vi "Control.AnalysisStop.vi"(11 "AnalysisRef":refnum<vi>) -> ()   [LabVIEW 2015, in "NIAnalysis.lvlib"]
uses:
  NIAnalysis.lvlib
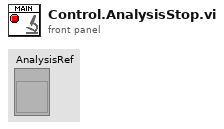
[diagram p1: front panel]
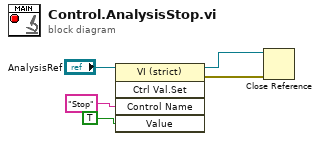
[diagram p0: block diagram]
diagram:
  n1 = invoke class="VI (strict)" method="Ctrl Val.Set"(reference="AnalysisRef", "Control Name"="Stop", "Value"=TRUE) -> (reference out=w3:refnum<vi>, error out=w4:errorcluster)  [unwired: 2 in, 3 out]
  n2 = Close Reference(reference=w3, error in (no error)=w4) -> ()  [unwired: 1 out]
